vi "Time to subscribe.vi"(8 "error in (no error)":errorcluster, 11 "Process Pulse in":refnum<class "Process Object.lvclass">) -> (0 "error out":errorcluster, 3 "Process Pulse out":refnum<class "Process Object.lvclass">)   [LabVIEW 2015, in "Process Object.lvclass"]
uses:
  Process Object.lvclass
  <vilib>/ActorFramework/Actor/Actor.lvclass/Actor.ctl
  <vilib>/ActorFramework/Message Enqueuer/Message Enqueuer.lvclass/Message Enqueuer.ctl
  Measure Object Messages/Subscribe Request Msg/Subscribe Request Msg.lvclass/Subscribe Request Msg.ctl
  Measure Object/Read Name.vi
  <vilib>/ActorFramework/Message Enqueuer/Init from Existing Queue.vi
  <vilib>/ActorFramework/Message Enqueuer/Enqueue.vi
  <vilib>/ActorFramework/Message Priority Queue/Priority Enqueue.vi
  Measure Object/Measure Object.lvclass
  <vilib>/ActorFramework/Message Enqueuer/Message Enqueuer.lvclass
  Measure Object Messages/Subscribe Request Msg/Subscribe Request Msg.lvclass
  <vilib>/ActorFramework/Actor/Actor.lvclass
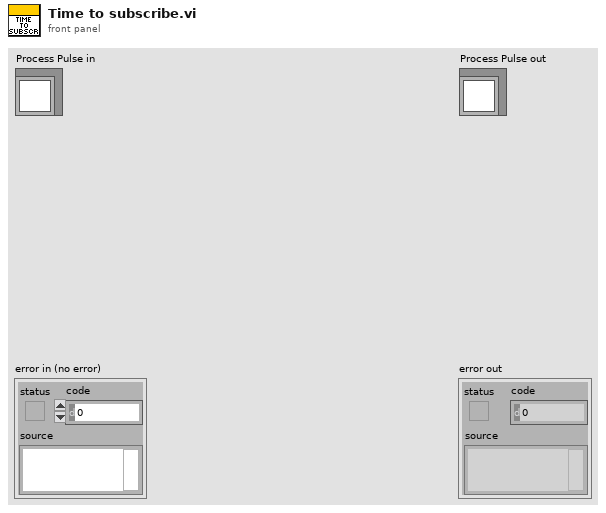
[diagram p1: front panel]
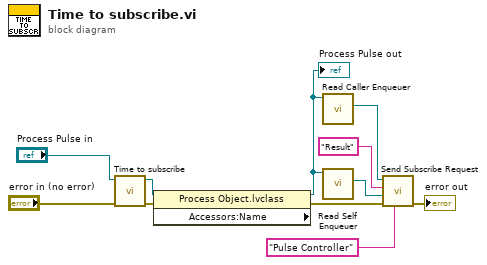
[diagram p0: block diagram]
diagram:
  n1 = call-parent "Time to subscribe.vi"("error in (no error)"="error in (no error)", "Measure Object in"="Process Pulse in") -> ("error out"=w4:errorcluster, "Measure Object out"=w5:refnum<class "Process Object.lvclass">)  [unwired: 8 in]
  n2 = property class="Process Object.lvclass" props=["Accessors:Name"](reference=w5, error in=w4) -> (reference out=w1:refnum<class "Process Object.lvclass">, error out=w7:errorcluster)  [unwired: 1 out]
  "Process Pulse out" <- w1
  n3 = call <vilib>:"Read Caller Enqueuer.vi"("Actor"=w1) -> ("Caller Enqueuer"=w6:refnum<class "Message Enqueuer.lvclass">)  [unwired: 10 in]
  n4 = call <vilib>:"Read Self Enqueuer.vi"("Actor"=w1) -> ("Self Enqueuer"=w8:refnum<class "Message Enqueuer.lvclass">)  [unwired: 10 in]
  n5 = call "Send Subscribe Request.vi"("Broadcaster"="Pulse Controller" ("Name"), "error in (no error)"=w7, "Subscriber Enqueuer"=w8, "Topic"="Result", "Message Enqueuer"=w6) -> ("error out"=→"error out":errorcluster)  [unwired: 5 in, 1 out]
